vi "报表表格.vi"() -> ()   [LabVIEW 2013]
uses:
  <vilib>/Utility/config.llb/NI_LVConfig.lvlib
panel:
  in  "油动机实验报告":T1
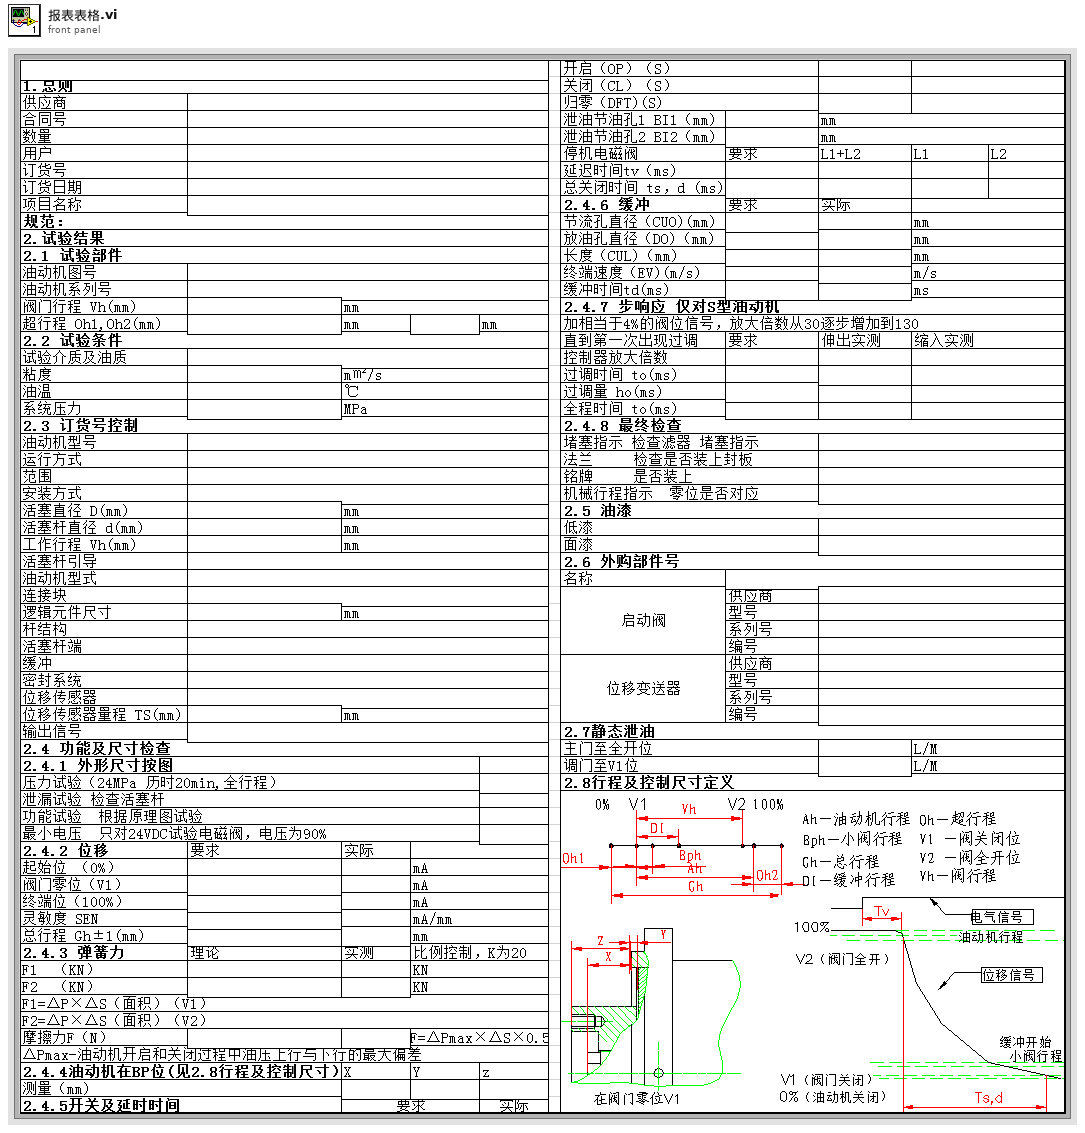
[diagram p1: front panel]
types:
  T1 = cluster{"油动机试验报告名称":string, "供应商1":string, "合同号1":string, "数量1":string, "用户1":string, "订货号1":string, "订货日期1":string, "项目名称1":string, "油动机图号2.1":string, "油动机系列号2.1":string, "阀门行程Vh":string, "试验介质及油质2.2":string, "超行程Oh1":string, "超行程Oh2":string, "粘度2.2":string, "油温2.2":string, "系统压力2.2":string, "油动机型号2.3":string, "运行方式2.3":string, "范围2.3":string, "安装方式2.3":string, "活塞直径D":string, "活塞杆直径d":string, "工作行程Vh2.3":string, "活塞杆引导2.3":string, "油动机型式2.3":string, "连接块2.3":string, "逻辑元件尺寸2.3":string, "杆结构2.3":string, "活塞杆端2.3":string, "缓冲2.3":string, "密封系统2.3":string, "位移传感器2.3":string, "位移传感器量程TS":string, "输出信号":string, "外形尺寸_2.4.1":string, "泄漏试验与否_2.4.1":string, "功能试验与否_2.4.1":string, "最小电压试验与否_2.4.1":string, "压力试验与否_2.4.1":string, "要求起始位2.4.2":string, "实际起始位":string, "要求总行程Gh2.4.2":string, "理论摩擦力F2.4.3":string, "要求灵敏度2.4.2":string, "理论F12.4.3":string, "要求终端位2.4.2":string, "要求阀门零位2.4.2":string, "理论F22.4.3":string, "实际阀门零位V1":string, "实际终端位V2":string, "实际灵敏度SEN":string, "实际总行程Gh":string, "实测F1":string, "实测F2":string, "实测F":string, "油动机在BP位_测量_X":string, "油动机在BP位_测量_Y":string, "油动机在BP位_测量_Z":string, "要求开关延时_开启2.4.5":string, "实际OP":string, "要求开关延时_关闭2.4.5":string, "实际CL":string, "要求开关延时_归零2.4.5":string, "实际DFT":string, "泄油节油孔1_BI1_2.4.5":string, "泄油节油孔2_BI2_2.4.5":string, "要求延迟时间tv_2.4.5":string, "要求总关闭时间ts_2.4.5":string, "要求_终端速度_2.4.6":string, "要求_长度_2.4.6":string, "要求_放油孔直径_2.4.6":string, "要求_节流孔直径_2.4.6":string, "延迟时间L1L2":string, "延迟时间L1":string, "延迟时间L2":string, "总关闭时间L1L2":string, "总关闭时间L1":string, "总关闭时间L2":string, "实际_节流孔直径_2.4.6":string, "缓冲时间td":string, "实际终端速度":string, "实际_长度_2.4.6":string, "实际_放油孔直径_2.4.6":string, "要求_缓冲时间_2.4.6":string, "控制器放大倍数_2.4.7":string, "伸出实测_控制器放大倍数_2.4.7":string, "缩入实测_控制器放大倍数_2.4.7":string, "要求_全程时间_2.4.7":string, "要求_过调时间_2.4.7":string, "要求_过调量_2.4.7":string, "伸出实测_全程时间":string, "伸出实测_过调量":string, "伸出实测_过调时间":string, "缩入实测_全程时间":string, "缩入实测_过调量":string, "缩入实测_过调时间":string, "堵塞指示_2.4.8":string, "法兰_2.4.8 ":string, "铭牌_2.4.8 ":string, "机械行程指示_2.4.8 ":string, "低漆_2.5":string, "面漆_2.5":string, "名称_2.6":string, "启动阀_供应商_2.6":string, "启动阀_型号_2.6":string, "启动阀_系列号_2.6":string, "启动阀_编号_2.6":string, "位移变送器_供应商_2.6":string, "位移变送器_型号_2.6":string, "位移变送器_系列号_2.6":string, "位移变送器_编号_2.6":string, "主门至全开位_2.7":string, "调门至V1位_2.7":string}
  T2 = typedef "NI_LVConfig.lvlib/Config Data RefNum.ctl" = refnum<k1>
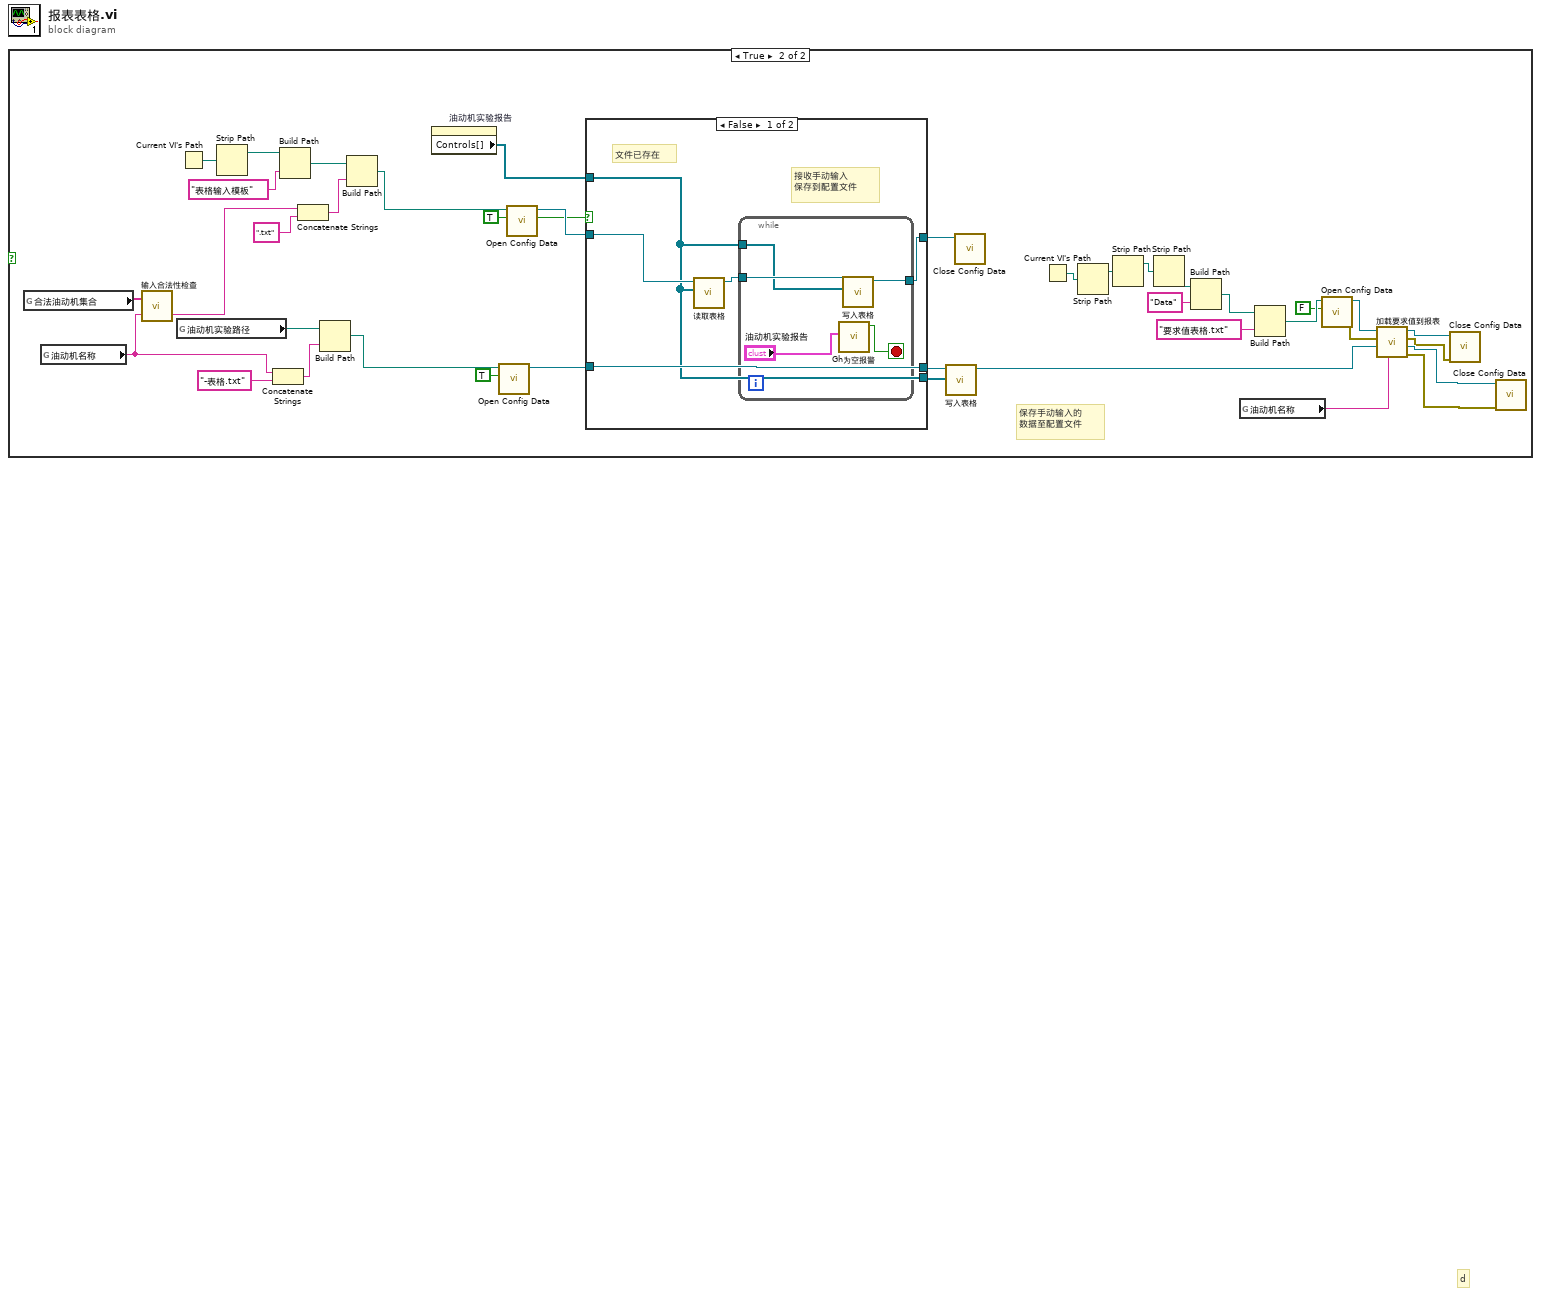
[diagram p0: block diagram]
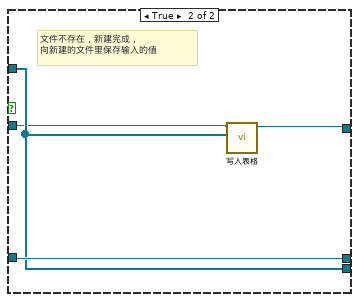
[diagram p3: hidden frame]
diagram:
  # "d"
  n1 = case shown="True" {
    selector: _ -> [_ _]
    frame False {
      # "E:\\testdir\\195-2\\GV7\\GV7\\GV7-1.2表格.txt"
    }
    frame True {
      # "保存手动输入的\n数据至配置文件"
      n2 = global read "合法油动机集合.vi" "合法油动机集合"() -> (w5:string[])
      n3 = global read "油动机名称.vi" "油动机名称"() -> (w4:string)
      n4 = call "输入合法性检查.vi"("被检查名称"=w4, "合法名称集合"=w5) -> ("合法名称"=w3:string)  [unwired: 1 out]
      n5 = global read "油动机实验路径.vi" "油动机实验路径"() -> (w6:path)
      n6 = Current VI's Path() -> (path=w37:path)
      n7 = Strip Path(path=w37) -> (stripped path=w36:path)  [unwired: 1 out]
      n8 = Concatenate Strings(w4, "-表格.txt" ("字符串")) -> (w38:string)
      n9 = Build Path(base path=w36, name or relative path="表格输入模板" ("名称或相对路径")) -> (appended path=w34:path)
      n10 = Concatenate Strings(w3, ".txt" ("字符串")) -> (w2:string)
      n11 = Build Path(base path=w6, name or relative path=w38) -> (appended path=w27:path)
      n12 = Build Path(base path=w34, name or relative path=w2) -> (appended path=w32:path)
      n13 = property on="油动机实验报告" class="Clust (strict)"() -> ("Controls[]"=w29:refnum<vi>[])  [unwired: 2 in, 2 out]
      n14 = call <vilib>:"Open Config Data.vi"("create file if necessary (T)"=TRUE, "configuration file path"=w27) -> ("refnum"=w25:T2)  [unwired: 7 in, 2 out]
      n15 = call <vilib>:"Open Config Data.vi"("create file if necessary (T)"=TRUE, "configuration file path"=w32) -> ("file created?"=w31:bool, "refnum"=w40:T2)  [unwired: 7 in, 1 out]
      n16 = case shown="False" w31 {
        tunnel: w40 -> [w45 w52]
        tunnel: w29 -> [w41 w53]
        tunnel: [w43 w51] -> w28
        tunnel: [w42 w54] -> w24
        tunnel: w25 -> [w42 w54]
        tunnel: [w41 w53] -> w23
        frame False {
          # "接收手动输入\n保存到配置文件"
          # "文件已存在"
          n17 = call "读取表格.vi"("Controls[]"=w41, "引用句柄输入"=w45) -> ("引用句柄输出"=w44:T2)  [unwired: 8 in, 1 out]
          n18 = while {
            tunnel: w44 -> [w50]
            tunnel: [w49] -> w43
            tunnel: w41 -> [w48]
            stop <- w46 stop-if-true
            n19 = call "Gh为空报警.vi"("油动机实验报告"="油动机实验报告") -> ("flag"=w46:bool)  [unwired: 9 in, 1 out]
            n20 = call "写入表格.vi"("Controls[]"=w48, "引用句柄输入"=w50) -> ("引用句柄输出"=w49:T2)  [unwired: 8 in, 1 out]
          }
        }
        frame True {
          # "文件不存在，新建完成，\n向新建的文件里保存输入的值"
          n21 = call "写入表格.vi"("Controls[]"=w53, "引用句柄输入"=w52) -> ("引用句柄输出"=w51:T2)  [unwired: 8 in, 1 out]
        }
      }
      n22 = call "写入表格.vi"("Controls[]"=w23, "引用句柄输入"=w24) -> ("引用句柄输出"=w22:T2)  [unwired: 8 in, 1 out]
      n23 = call <vilib>:"Close Config Data.vi"("refnum"=w28) -> ()  [unwired: 9 in, 2 out]
      n24 = Current VI's Path() -> (path=w12:path)
      n25 = Strip Path(path=w12) -> (stripped path=w14:path)  [unwired: 1 out]
      n26 = Strip Path(path=w14) -> (stripped path=w15:path)  [unwired: 1 out]
      n27 = Strip Path(path=w15) -> (stripped path=w16:path)  [unwired: 1 out]
      n28 = Build Path(base path=w16, name or relative path="Data" ("名称或相对路径")) -> (appended path=w13:path)
      n29 = global read "油动机名称.vi" "油动机名称"() -> (w1:string)
      n30 = Build Path(base path=w13, name or relative path="要求值表格.txt" ("名称或相对路径")) -> (appended path=w19:path)
      n31 = call <vilib>:"Open Config Data.vi"("create file if necessary (T)"=FALSE, "configuration file path"=w19) -> ("error out"=w9:errorcluster, "refnum"=w10:T2)  [unwired: 7 in, 1 out]
      n32 = call "加载要求值到报表.vi"("油动机名称"=w1, "试验表格refnum in"=w22, "错误输入（无错误）"=w9, "要求值表格refnum in"=w10) -> ("error out"=w20:errorcluster, "试验表格refnum out"=w21:T2, "错误输出"=w7:errorcluster, "要求值表格refnum out"=w8:T2)  [unwired: 4 in]
      n33 = call <vilib>:"Close Config Data.vi"("error in (no error)"=w7, "refnum"=w8) -> ()  [unwired: 8 in, 2 out]
      n34 = call <vilib>:"Close Config Data.vi"("error in (no error)"=w20, "refnum"=w21) -> ()  [unwired: 8 in, 2 out]
    }
  }
